vi "testDriver.vi"() -> ()   [LabVIEW 2012]
uses:
  <vilib>/DAQmx/configure/timing.llb/DAQmx Timing (Implicit).vi
  <resource>/objmgr/daqmx.rc
panel:
  out "pulse 1/2 len (ms)":dbl
  in  "Meter":dbl(knob) scale=0.0..49.0
  out "mm/s (timed)":dbl
  in  "Run":bool
  in  "travel dist(mm)":i32=100
  in  "Direction":bool
  in  "enable":bool
  # "=17400 to go across"
  # "0.0001"
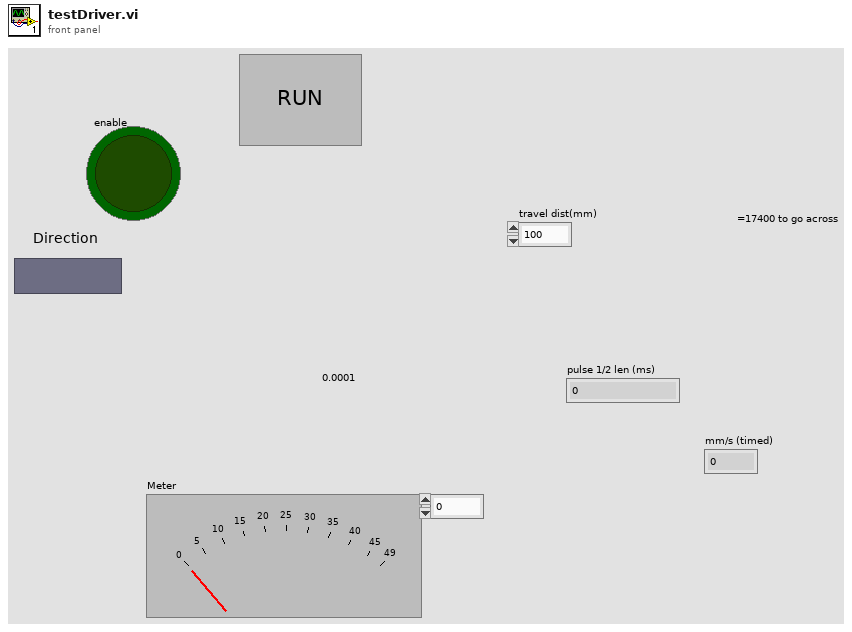
[diagram p1: front panel]
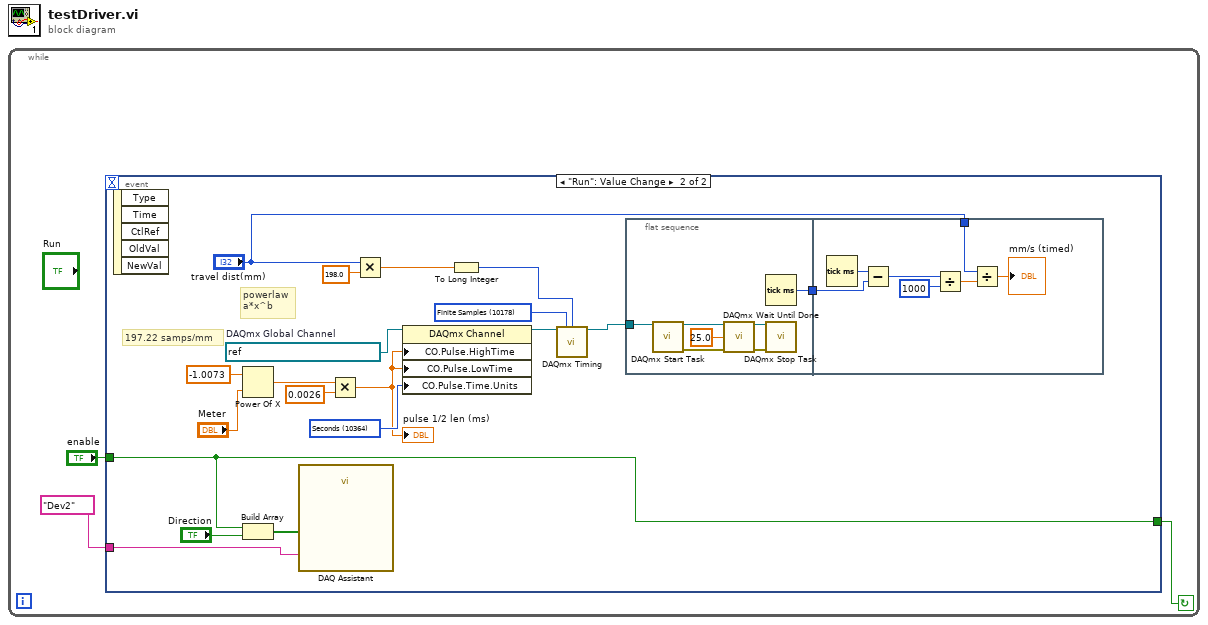
[diagram p0: block diagram]
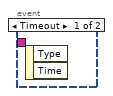
[diagram p2: hidden frame]
diagram:
  n1 = while {
    stop <- w2 continue-if-true
    n2 = event shown="[1] \"Run\": Value Change" {
      selector: _ -> [_ _]
      dyn-events: _ -> [_ _]
      timeout: _ -> [_ _]
      tunnel: tag "Dev2" ("device name") -> [_ w17]
      tunnel: [_ w14] -> w2
      tunnel: "enable" -> [_ w14]
      event Timeout {
        n3 = event-data() -> ()  [unwired: 1 in, 2 out]
      }
      event "Run": Value Change {
        w22 = 10364 items=["Seconds"=10364] ("CO.Pulse.Time.Units")
        w19 = 10178 items=["Finite Samples"=10178, "Continuous Samples"=10123, "Hardware Timed Single Point"=12522] ("sample mode")
        w18 = refnum<k21> "MyPulseOutputChannel"  # DAQmx Global Channel
        # "powerlaw\na*x^b"
        # "197.22 samps/mm"
        n4 = event-data() -> ()  [unwired: 1 in, 5 out]
        n5 = Power Of X(1:"Meter", 2:-1.0073) -> (0:w6:dbl)
        n6 = Build Array(w14, "Direction") -> (w15:bool[])
        n7 = call "DAQ Assistant"("data"=w15, "device name"=w17) -> ()  [unwired: 16 in, 2 out]
        n8 = Multiply(x=w6, y=0.0026) -> (x*y=w4:dbl)
        "pulse 1/2 len (ms)" <- w4
        n9 = Multiply(x="travel dist(mm)", y=198.0) -> (x*y=w12:dbl)
        n10 = property class="DAQmx Channel"(reference=w18, "CO.Pulse.HighTime"=w4, "CO.Pulse.LowTime"=w4, "CO.Pulse.Time.Units"=w22) -> (reference out=w21:refnum<k21>)  [unwired: 1 in, 1 out]
        n11 = To Long Integer(number=w12) -> (32bit integer=w11:i32)
        n12 = call-poly <vilib>:"DAQmx Timing.vi"("task/channels in"=w21, "sample mode"=w19, "samples per channel"=w11) -> ("task out"=w20:refnum<k21>)  [unwired: 11 in, 1 out]
        n13 = flat-sequence {
          tunnel: w20 -> [w27]
          tunnel: [w23] -> w10
          tunnel: w10 -> [w36]
          tunnel: "travel dist(mm)" -> [w32]
          frame #0 {
            n14 = call <vilib>:"DAQmx Start Task.vi"("task/channels in"=w27) -> ("task out"=w28:refnum<k21>, "error out"=w25:errorcluster)  [unwired: 13 in]
            n15 = call <vilib>:"DAQmx Wait Until Done.vi"("task/channels in"=w28, "timeout (sec)"=25.0, "error in"=w25) -> ("task out"=w26:refnum<k21>, "error out"=w24:errorcluster)  [unwired: 11 in]
            n16 = Tick Count (ms)() -> (millisecond timer value=w23:u32)
            n17 = call <vilib>:"DAQmx Stop Task.vi"("task/channels in"=w26, "error in"=w24) -> ()  [unwired: 12 in, 2 out]
          }
          frame #1 {
            n18 = Tick Count (ms)() -> (millisecond timer value=w35:u32)
            n19 = Subtract(x=w35, y=w36) -> (x-y=w34:u32)
            n20 = Divide(x=w34, y=u32 1000) -> (x/y=w31:dbl)
            n21 = Divide(x=w32, y=w31) -> (x/y=→"mm/s (timed)":dbl)
          }
        }
      }
    }
  }
